vi "Handle Command.vi"(8 "error in (no error)":errorcluster, 9 "Value":bool, 11 "Valve in":refnum<class "LimitControl.lvclass">) -> (0 "error out":errorcluster, 3 "Valve out":refnum<class "LimitControl.lvclass">)   [LabVIEW 2020, in "VolatusControl.lvlib" / "LimitControl.lvclass"]
uses:
  LimitControl.lvclass
  LimitControl.lvclass/LimitControl.ctl
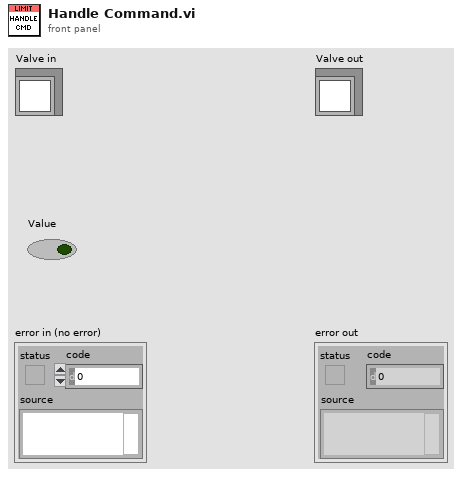
[diagram p1: front panel]
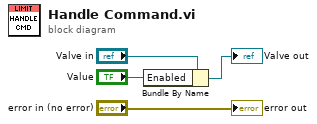
[diagram p0: block diagram]
diagram:
  n1 = Bundle By Name(cluster="Valve in", "Enabled"="Value") -> (→"Valve out":refnum<class "LimitControl.lvclass">)
  "error out" <- "error in (no error)"
